vi "File_IO.vi"() -> ()   [LabVIEW 2018]
uses:
  <vilib>/Utility/file.llb/Write Delimited Spreadsheet (I64).vi
  <vilib>/measure/NI_MABase.lvlib
panel:
  out "데이터":waveform(dbl)[](graph)
  out "레코드":errorcluster[](array[cluster])
  in  "카운트(1)":i32
  in  "정지 2":bool
  in  "정지":bool
  out "배열 2":i32[][](array[numeric])
  out "배열":i32[](array[numeric])
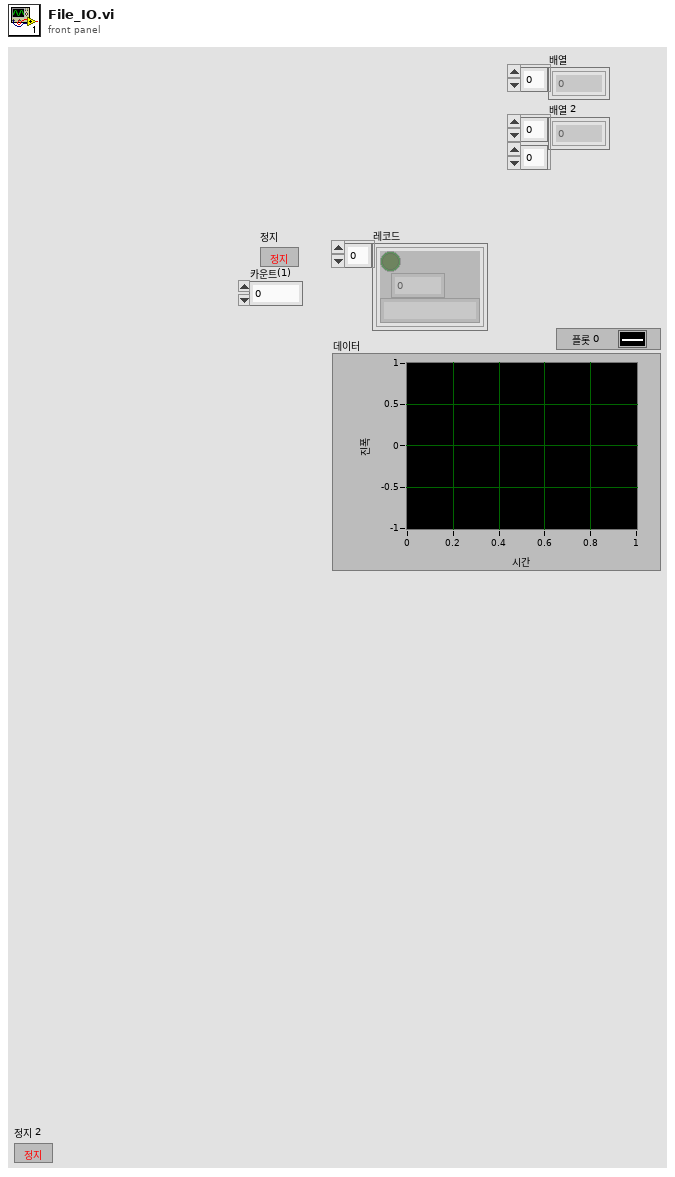
[diagram p1: front panel]
types:
  T1 = enum16{"open", "open or create", "create or replace", "create", "open (read-only)"}
  T2 = enum16{"Sine Wave", "Triangle Wave", "Square Wave", "Sawtooth Wave"}
  T3 = enum16{"open", "replace", "create", "open or create", "replace or create", "replace or create with confirmation"}
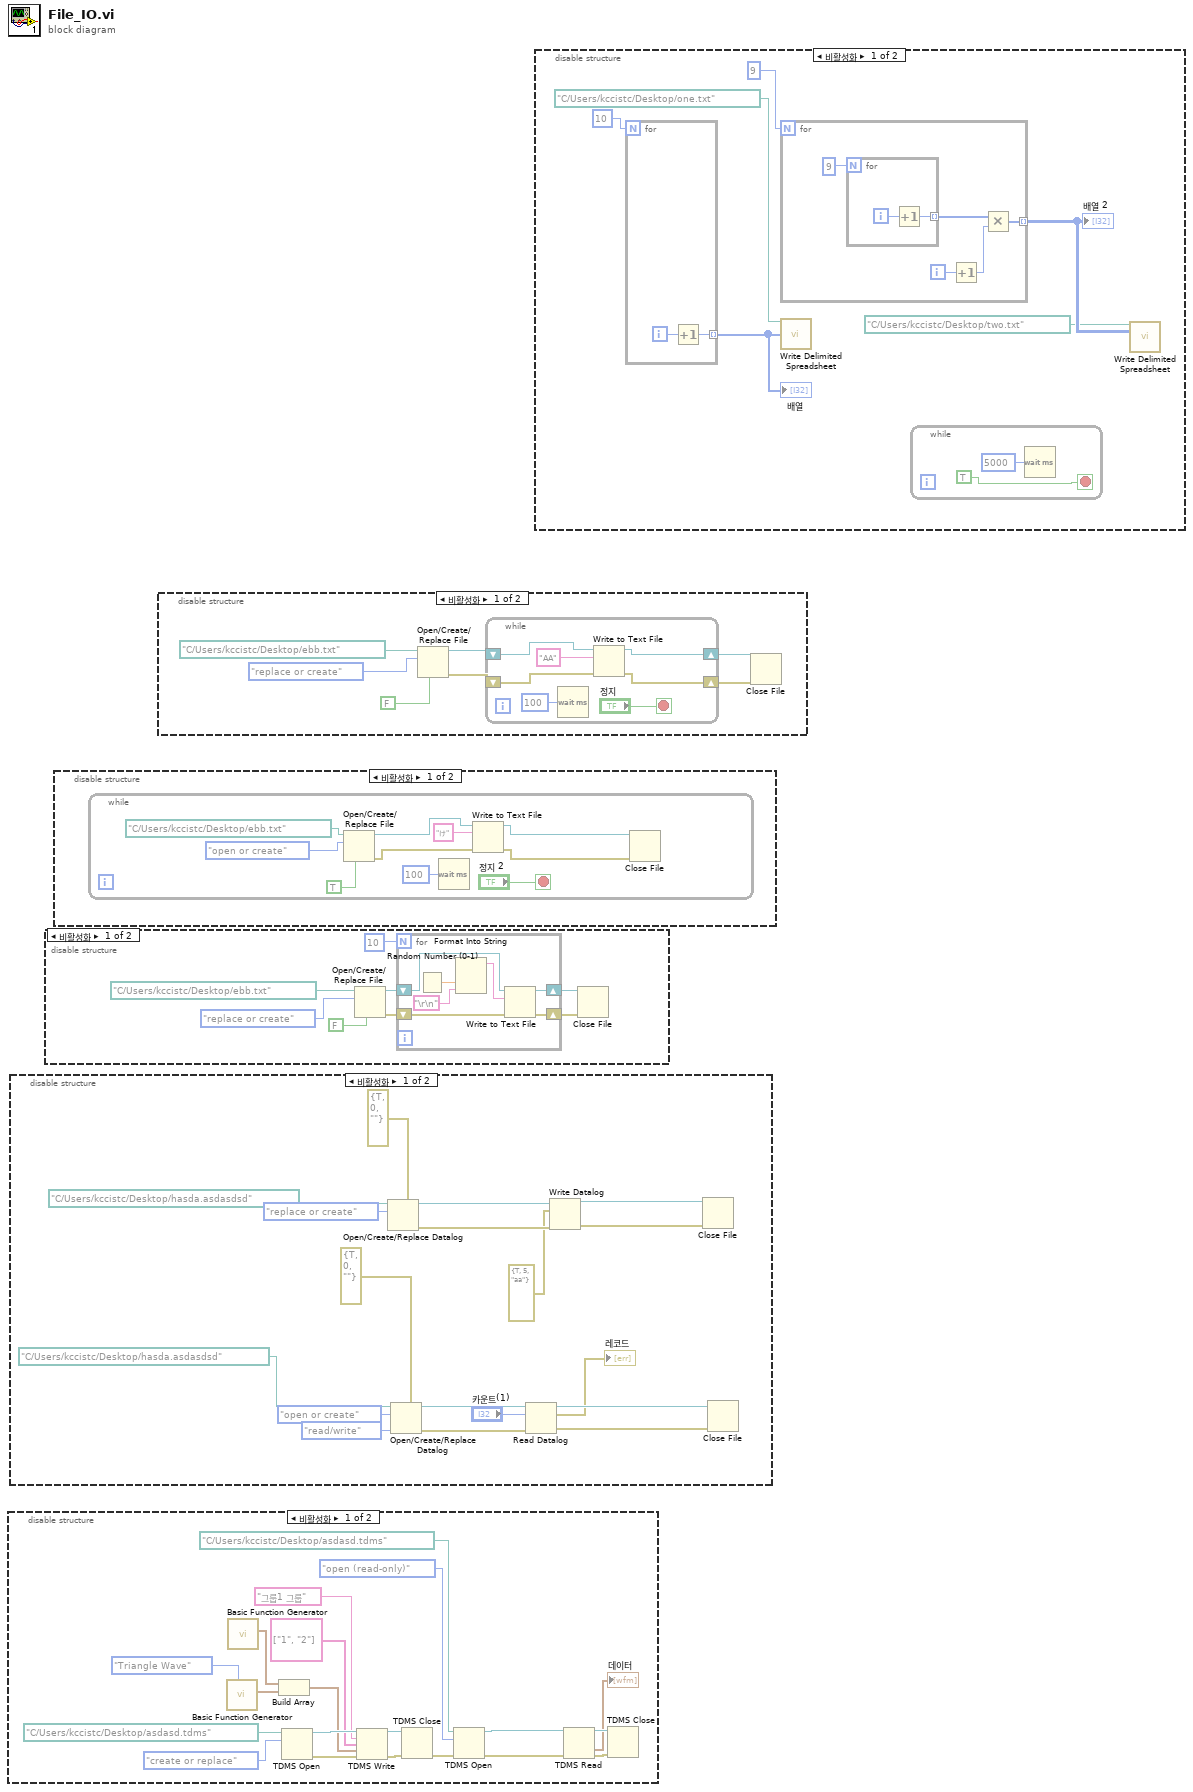
[diagram p0: block diagram]
diagram:
  n1 = disable-structure shown="비활성화" {
    frame Disabled {
      n2 = call <vilib>:"Basic Function Generator.vi"("signal type"=T2."Triangle Wave") -> ("signal out"=w13:waveform(dbl))  [unwired: 8 in, 2 out]
      n3 = call <vilib>:"Basic Function Generator.vi"() -> ("signal out"=w12:waveform(dbl))  [unwired: 9 in, 2 out]
      n4 = Build Array(w12, w13) -> (w11:waveform(dbl)[])
      n5 = TDMS Open(10:T1."create or replace" ("동작(0:open)"), 11:path "C:/Users/kccistc/Desktop/asdasd.tdms" ("파일 경로(대화 상자 사용)")) -> (0:w18:errorcluster, 3:w19:refnum<k34>)  [unwired: 5 in]
      n6 = TDMS Write(0:w19, 5:"그룹1 그룹" ("그룹 이름 입력(제목없음)"), 7:string[] ["1", "2"] ("채널 이름 입력(제목없음)"), 9:w11, 11:w18) -> (4:w17:refnum<k34>, 15:w16:errorcluster)  [unwired: 1 in, 2 out]
      n7 = TDMS Close(8:w16, 11:w17) -> (0:w1:errorcluster)  [unwired: 1 out]
      n8 = TDMS Open(8:w1, 10:T1."open (read-only)" ("동작(0:open)"), 11:path "C:/Users/kccistc/Desktop/asdasd.tdms" ("파일 경로(대화 상자 사용)")) -> (0:w5:errorcluster, 3:w6:refnum<k34>)  [unwired: 4 in]
      n9 = TDMS Read(0:w6, 11:w5) -> (4:w4:refnum<k34>, 10:→"데이터":waveform(dbl)[], 15:w3:errorcluster)  [unwired: 6 in, 3 out]
      n10 = TDMS Close(8:w3, 11:w4) -> ()  [unwired: 2 out]
    }
    frame Enabled {
    }
  }
  n11 = disable-structure shown="비활성화" {
    frame Disabled {
      n12 = Open/Create/Replace Datalog(5:errorcluster {TRUE, 0, ""}, 10:T3."replace or create" ("동작(0:open)"), 11:path "C:/Users/kccistc/Desktop/hasda.asdasdsd" ("데이터로그 경로(대화 상자 사용)")) -> (0:w35:errorcluster, 3:w38:refnum<k1>)  [unwired: 3 in, 1 out]
      n13 = Open/Create/Replace Datalog(5:errorcluster {TRUE, 0, ""}, 9:enum16{"read/write", "read-only", "write-only"}."read/write" ("접근(0:read/write)"), 10:T3."open or create" ("동작(0:open)"), 11:path "C:/Users/kccistc/Desktop/hasda.asdasdsd" ("데이터로그 경로(대화 상자 사용)")) -> (0:w34:errorcluster, 3:w32:refnum<k1>)  [unwired: 2 in, 1 out]
      n14 = Read Datalog(4:w34, 6:"카운트(1)", 7:w32) -> (0:w33:errorcluster, 2:→"레코드":errorcluster[], 3:w31:refnum<k1>)
      n15 = Write Datalog(4:w35, 6:errorcluster {TRUE, 5, "aa"}, 7:w38) -> (0:w36:errorcluster, 3:w37:refnum<k1>)
      n16 = Close File(refnum=w37, error in=w36) -> ()  [unwired: 2 out]
      n17 = Close File(refnum=w31, error in=w33) -> ()  [unwired: 2 out]
    }
    frame Enabled {
    }
  }
  n18 = disable-structure shown="비활성화" {
    frame Disabled {
      n19 = Open/Create/Replace File(file path (use dialog)=path "C:/Users/kccistc/Desktop/ebb.txt" ("파일 경로(대화 상자 사용)"), operation (0:open)=T3."replace or create" ("동작(0:open)"), disable buffering (F)=FALSE ("버퍼링 비활성화(거짓)")) -> (refnum out=w43:refnum<file>, error out=w42:errorcluster)  [unwired: 3 in, 1 out]
      n20 = for {
        N: 10 -> [_]
        shift-right: [w53] -> w40
        shift-left: w42 -> [w50]
        shift-right: [w52] -> w41
        shift-left: w43 -> [w51]
        n21 = Random Number (0-1)() -> (number: 0 to 1=w48:dbl)
        n22 = Format Into String(w48, "\r\n") -> (resulting string=w47:string)  [unwired: 3 in, 1 out]
        n23 = Write to Text File(file (use dialog)=w51, text=w47, error in=w50) -> (refnum out=w52:refnum<file>, error out=w53:errorcluster)  [unwired: 1 in, 1 out]
      }
      n24 = Close File(refnum=w41, error in=w40) -> ()  [unwired: 2 out]
    }
    frame Enabled {
    }
  }
  n25 = disable-structure shown="비활성화" {
    frame Disabled {
      n26 = while {
        stop <- "정지 2" stop-if-true
        n27 = Open/Create/Replace File(file path (use dialog)=path "C:/Users/kccistc/Desktop/ebb.txt" ("파일 경로(대화 상자 사용)"), operation (0:open)=T3."open or create" ("동작(0:open)"), disable buffering (F)=TRUE ("버퍼링 비활성화(거짓)")) -> (refnum out=w60:refnum<file>, error out=w61:errorcluster)  [unwired: 3 in, 1 out]
        n28 = Wait (ms)(milliseconds to wait=u32 100 ("대기 시간 (ms)")) -> ()  [unwired: 1 out]
        n29 = Write to Text File(file (use dialog)=w60, text="け", error in=w61) -> (refnum out=w59:refnum<file>, error out=w58:errorcluster)  [unwired: 1 in, 1 out]
        n30 = Close File(refnum=w59, error in=w58) -> ()  [unwired: 2 out]
      }
    }
    frame Enabled {
    }
  }
  n31 = disable-structure shown="비활성화" {
    frame Disabled {
      n32 = Open/Create/Replace File(file path (use dialog)=path "C:/Users/kccistc/Desktop/ebb.txt" ("파일 경로(대화 상자 사용)"), operation (0:open)=T3."replace or create" ("동작(0:open)"), disable buffering (F)=FALSE ("버퍼링 비활성화(거짓)")) -> (refnum out=w67:refnum<file>, error out=w68:errorcluster)  [unwired: 3 in, 1 out]
      n33 = while {
        shift-right: [w75] -> w65
        shift-left: w68 -> [w72]
        shift-right: [w74] -> w66
        shift-left: w67 -> [w73]
        stop <- "정지" stop-if-true
        n34 = Wait (ms)(milliseconds to wait=u32 100 ("대기 시간 (ms)")) -> ()  [unwired: 1 out]
        n35 = Write to Text File(file (use dialog)=w73, text="AA", error in=w72) -> (refnum out=w74:refnum<file>, error out=w75:errorcluster)  [unwired: 1 in, 1 out]
      }
      n36 = Close File(refnum=w66, error in=w65) -> ()  [unwired: 2 out]
    }
    frame Enabled {
    }
  }
  n37 = disable-structure shown="비활성화" {
    frame Disabled {
      n38 = for {
        N: 10 -> [_]
        tunnel: [w93] -> w82 mode=indexing
        i -> [w94]
        n39 = Increment(x=w94) -> (x+1=w93:i32)
      }
      "배열" <- w82
      n40 = for {
        N: 9 -> [_]
        tunnel: [w86] -> w80 mode=indexing
        i -> [w89]
        n41 = for {
          N: 9 -> [_]
          tunnel: [w91] -> w88 mode=indexing
          i -> [w92]
          n42 = Increment(x=w92) -> (x+1=w91:i32)
        }
        n43 = Increment(x=w89) -> (x+1=w87:i32)
        n44 = Multiply(x=w88, y=w87) -> (x*y=w86:i32[])
      }
      "배열 2" <- w80
      n45 = call-poly <vilib>:"Write Delimited Spreadsheet.vi"("file path (dialog if empty)"=path "C:/Users/kccistc/Desktop/one.txt", "1D data"=w82) -> ()  [unwired: 12 in, 2 out]
      n46 = while {
        stop <- TRUE stop-if-true
        n47 = Wait (ms)(milliseconds to wait=u32 5000 ("대기 시간 (ms)")) -> ()  [unwired: 1 out]
      }
      n48 = call-poly <vilib>:"Write Delimited Spreadsheet.vi"("file path (dialog if empty)"=path "C:/Users/kccistc/Desktop/two.txt", "2D data"=w80) -> ()  [unwired: 12 in, 2 out]
    }
    frame Enabled {
    }
  }
